vi "Decimate Force curve.vi"(0 "Fcurve":T1, 1 "decimating factor":i32=1, 5 "error in (no error)":errorcluster) -> (14 "Decimated Fcurve":cluster{"X":dbl[], "Y":dbl[]}[](array[cluster]), 19 "error out":errorcluster)   [LabVIEW 2019, in "XYgraph.lvclass"]
doc: "Decimates the approach contact and retract by a decimating factor"
uses:
  XYgraph.lvclass
  Force Curve_tdms_class/Force Curve data.ctl
  <vilib>/Analysis/2dsp.llb/Decimate (single shot, DBL).vi
  <vilib>/Analysis/NI_AALPro.lvlib
  Force Curve_tdms_class/Force Curve_tdms.lvclass
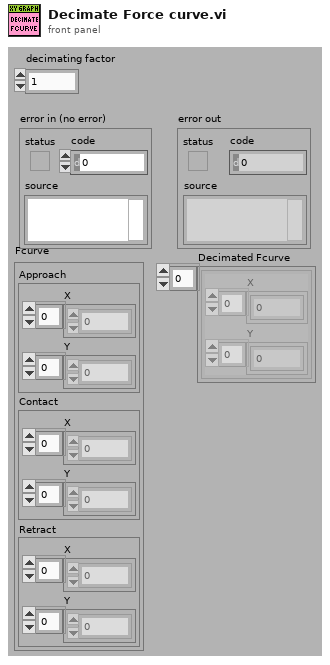
[diagram p1: front panel]
types:
  T1 = typedef "Force Curve_tdms.lvclass/Force Curve data.ctl" = cluster{"Approach":cluster{"X":dbl[], "Y":dbl[]}, "Contact":cluster{"X":dbl[], "Y":dbl[]}, "Retract":cluster{"X":dbl[], "Y":dbl[]}}
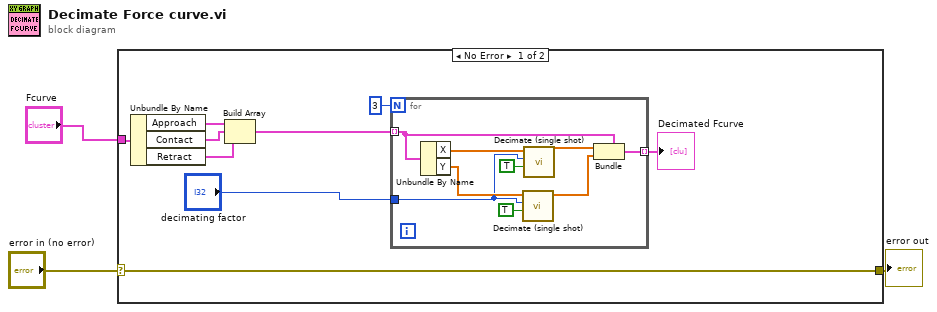
[diagram p0: block diagram]
diagram:
  n1 = case shown="No Error" "error in (no error)" {
    selector: "error in (no error)" -> [w12 w22]
    tunnel: [w12 w22] -> w2
    tunnel: "Fcurve" -> [w5 _]
    frame No Error {
      n2 = Unbundle By Name(w5) -> ("Approach"=w10:cluster{"X":dbl[], "Y":dbl[]}, "Contact"=w9:cluster{"X":dbl[], "Y":dbl[]}, "Retract"=w8:cluster{"X":dbl[], "Y":dbl[]})
      n3 = Build Array(w10, w9, w8) -> (w7:cluster{"X":dbl[], "Y":dbl[]}[])
      n4 = for {
        N: 3 -> [_]
        tunnel: w7 -> [w13] mode=indexing
        tunnel: "decimating factor" -> [w17]
        tunnel: [w14] -> w4 mode=indexing
        n5 = Unbundle By Name(w13) -> ("X"=w21:dbl[], "Y"=w20:dbl[])
        n6 = call-poly <vilib>:"Decimate (single shot).vi"("averaging"=TRUE, "decimating factor"=w17, "X"=w20) -> ("Decimated Array"=w15:dbl[])  [unwired: 7 in, 1 out]
        n7 = call-poly <vilib>:"Decimate (single shot).vi"("averaging"=TRUE, "decimating factor"=w17, "X"=w21) -> ("Decimated Array"=w16:dbl[])  [unwired: 7 in, 1 out]
        n8 = Bundle(cluster=w13, "X"=w16, "Y"=w15) -> (w14:cluster{"X":dbl[], "Y":dbl[]})
      }
      "Decimated Fcurve" <- w4
    }
    frame Error {
    }
  }
  "error out" <- w2
